vi "PS Control.vi"() -> ()   [LabVIEW 2025]
panel:
  in  "Stop":bool
  out "Tppms":dbl=378.0
  in  "set T":dbl=10.0
  in  "rate T":dbl=5.0 min=0.01 max=20.0
  in  "Setpoint [T]":dbl
  in  "Slew Rate [T/min]":dbl=0.3
  in  "T control":bool=TRUE
  in  "H control":bool=TRUE
  out "Field [T]":dbl=3.0
  out "helium level":bool
  out "LHe level":dbl=81.5
  out "error out":errorcluster
  out "Chamber\nStatus":i32(ring)=1 items=["ChamberUnknown"=0, "PurgedAndSealed"=1, "VentedAndSealed"=2, "Sealed"=3, "Purging"=4, "Venting"=5, "PreHiVac"=6, "HighVac"=7, "PumpContinuous"=8, "VentContinuous"=9, "ChamberFailure"=15]
  in  "set chamber":T1(ring)
  in  "shutdown":bool
  out "Field\nStatus":i32(ring)=4 items=["MagnetUnknown"=0, "StablePersistent"=1, "WarmingSwitch"=2, "CoolingSwitch"=3, "StableDriven"=4, "Iterating"=5, "Charging"=6, "Discharging"=7, "CurrentError"=8, "MagnetFailure"=15]
  out "Temperature\nStatus":i32(ring)=1 items=["TemperatureUnknown"=0, "Stable"=1, "Tracking"=2, "Near"=5, "Chasing"=6, "Filling"=7, "Standby"=10, "Disabled"=13, "ImpedanceNotFunction"=14, "TempFailure"=15]
  in  "LHe limit":dbl=60.0
  in  "resend chamber command":bool
  in  "Force High Vacuum":bool
  in  "HiVac pressure limit":dbl=0.0001 format="%#_4e"
  out "Position":dbl
  in  "Use rototar":bool
  in  "New position":dbl
  in  "Speed":dbl=5.0
  out "Pressure (Torr)":dbl=-1.0 format="%#_6e"
  in  "Mode":i32(ring) items=["Persistent", "Driven"]
  in  "Host (PPMS) computer name (or IP address)":string="SCM7"
  in  "port number":u16=3363
  # "(K/min)"
  # "Scroll down for a brief instruction."
  # "Error 56 or 63: Network error\n Possible reasons other than the obvious reasons (no internet, wrong host name, ...)\n   If the server program (PS Control.vi) is running under the development environment -> Check VI server settings (TCP/IP, port number, machine access).\n   If the server program is running under the run-time engine (.exe program) --> Check port number in the LV PPMS.ini file.\n  Try a different but similar port number.  \n Firewall issue on the host computer (rare) -> contact the computer support group.\n\nError 1004: server program not found (problem is at the host computer)\n Server program (PS Control.vi) is not running on the PPMS computer.  --> Start the server program.\n If the server program does not start, try to start it under a different mode (administrator or non-admininstrator). The server program will not start  unless it starts with the same mode with the PPMS multivu program.\n\nHow to use. \n\nFor  NML Data Acqustion.vi. (1) select 'Field' to read the field value, (2) select 'VI server read' to read the temperature (VI name: PS Control.vi, Control name: Tppms)\nFor LowMaster.vi, use the VI server menu to change the temperature, field and the other settings of the PPMS.\nFor MonoVu, use the built-in menu to control the field/temperature and the VI server menu to change the other settings of the PPMS."
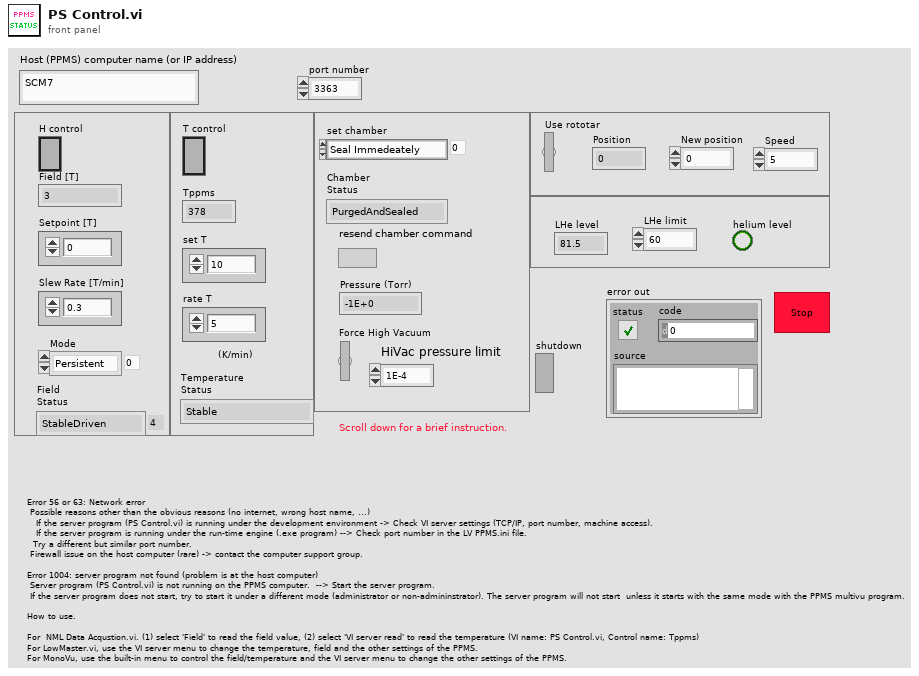
[diagram p1: front panel]
types:
  T1 = enum16{"Seal Immedeately", "Purge and Seal", "Vent and Seal", "Pump continuously", "Vent continuously", "HighVac"}
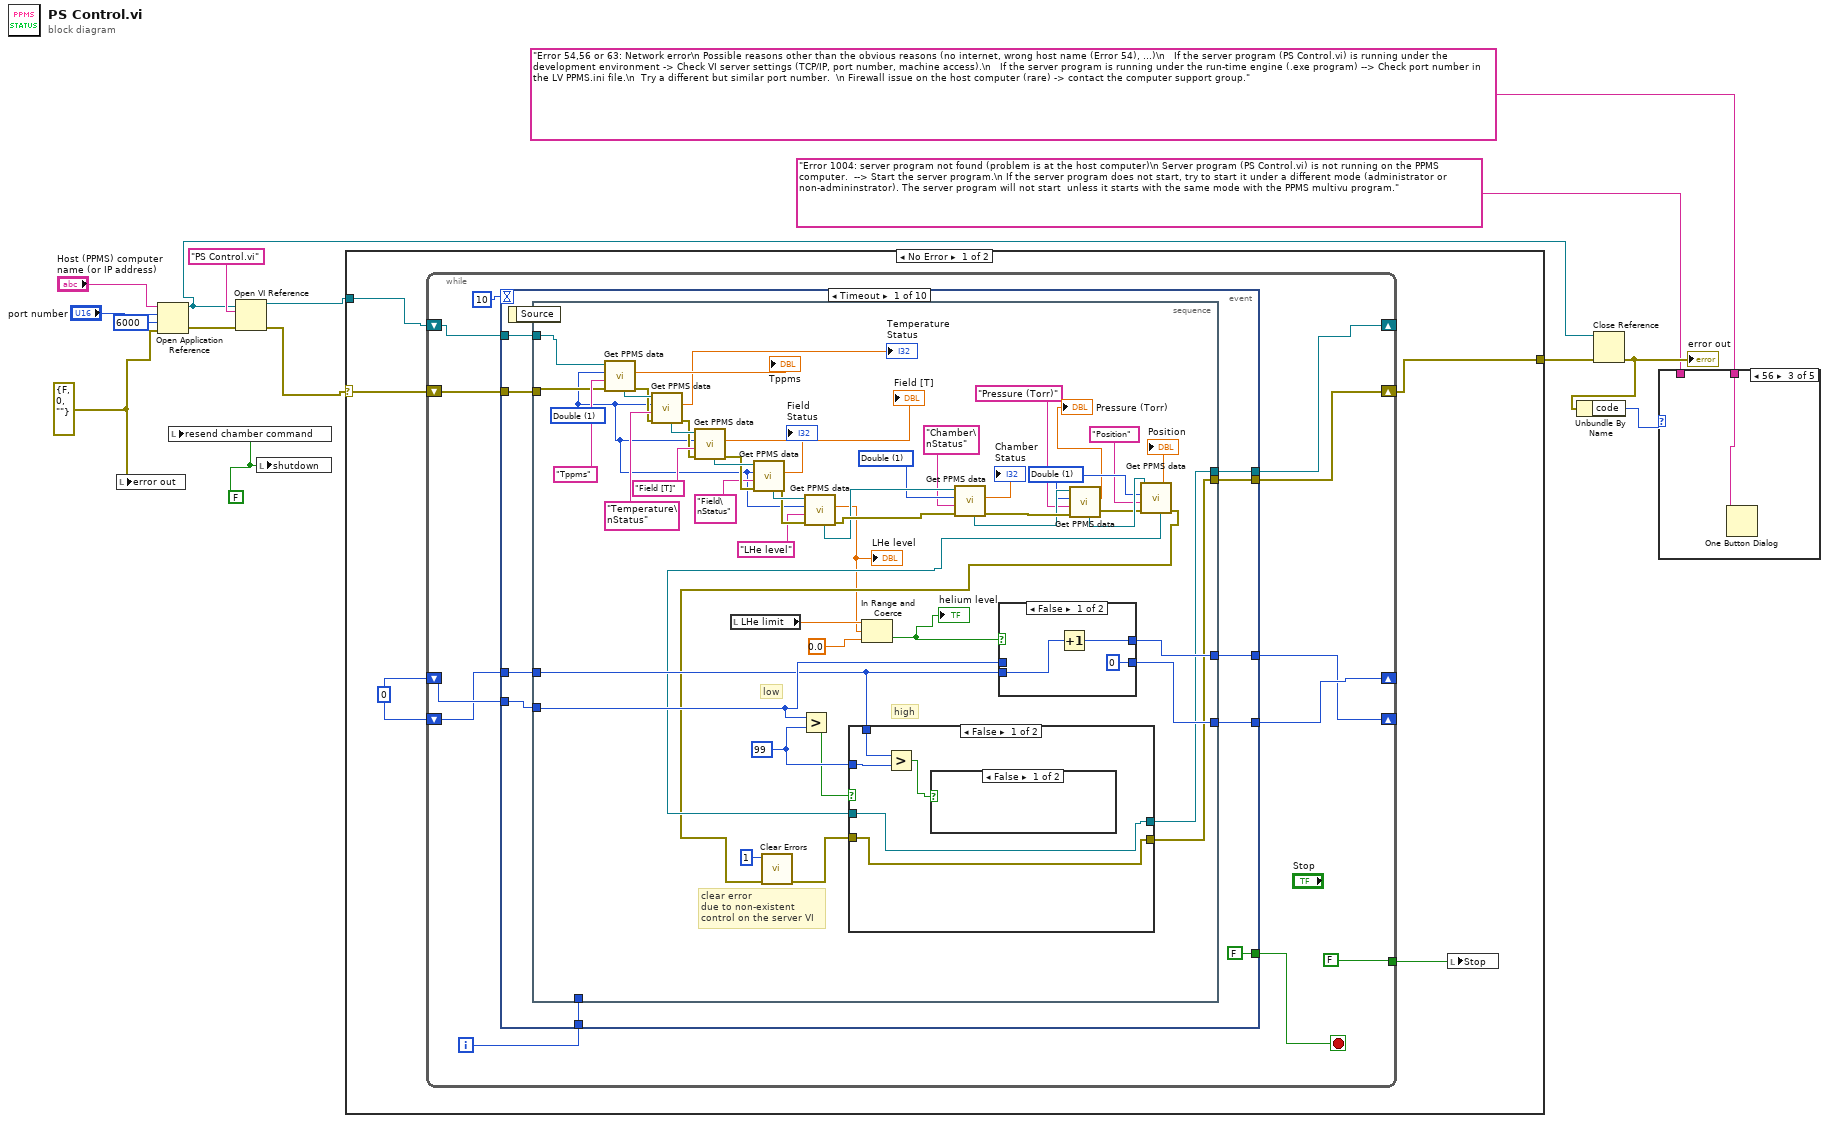
[diagram p0: block diagram]
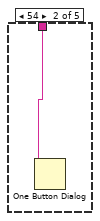
[diagram p3: hidden frame]
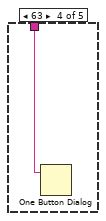
[diagram p4: hidden frame]
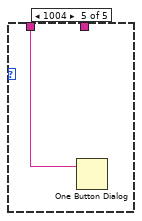
[diagram p5: hidden frame]
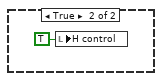
[diagram p6: hidden frame]
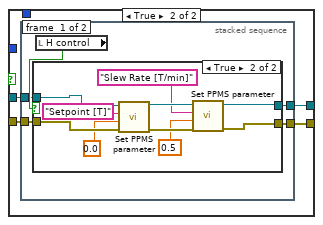
[diagram p7: hidden frame]
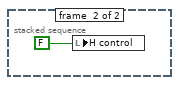
[diagram p9: hidden frame]
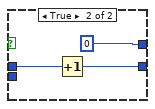
[diagram p10: hidden frame]
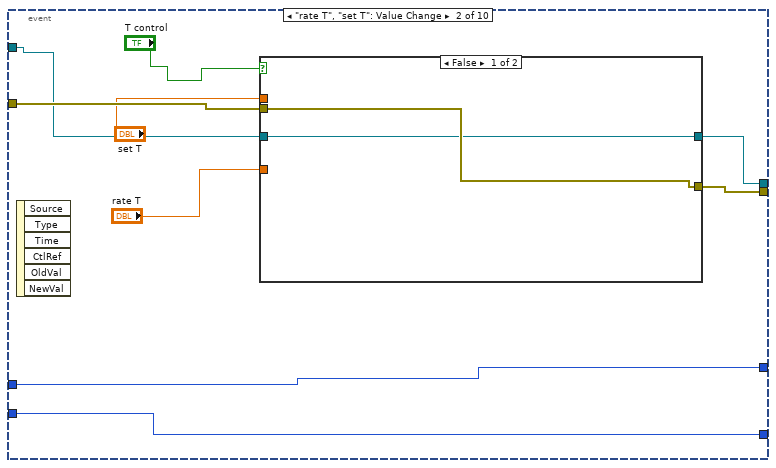
[diagram p11: hidden frame]
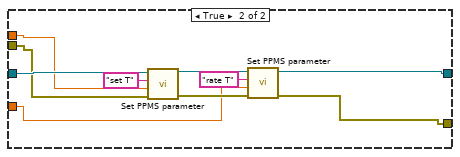
[diagram p12: hidden frame]
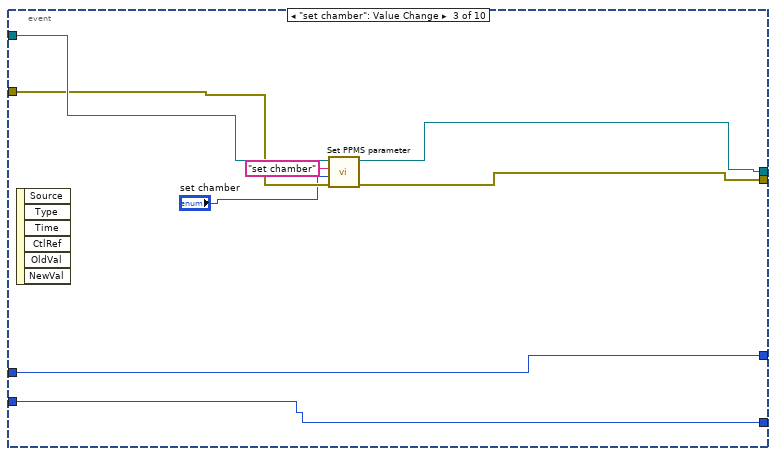
[diagram p13: hidden frame]
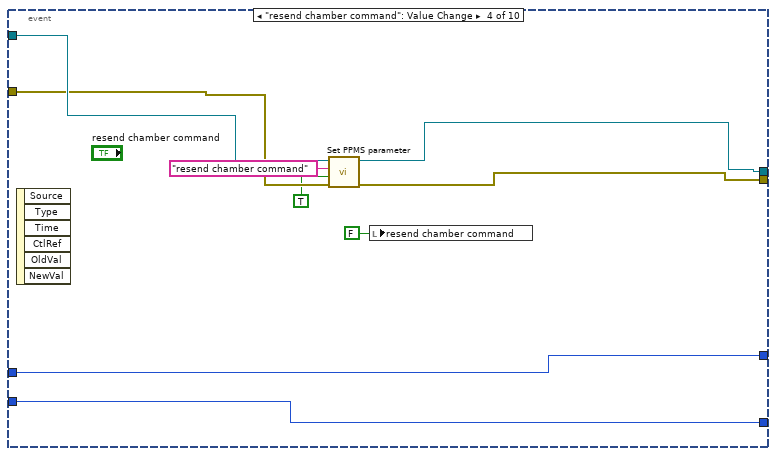
[diagram p14: hidden frame]
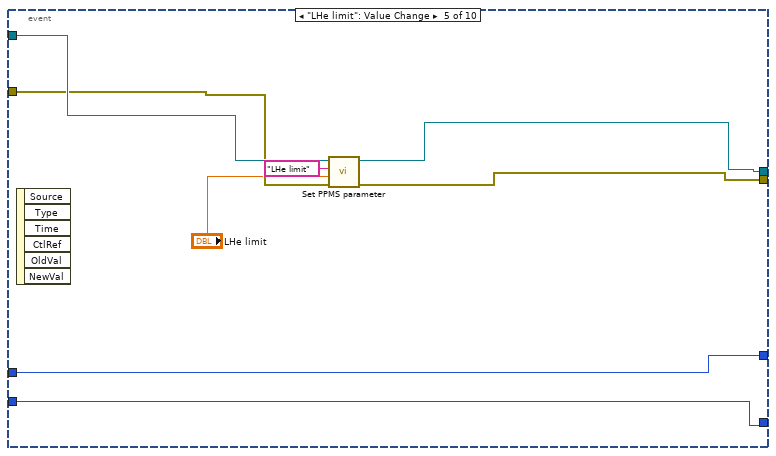
[diagram p15: hidden frame]
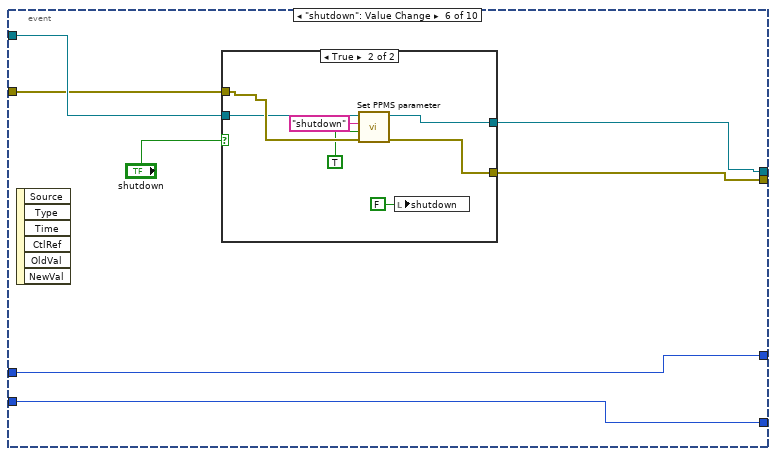
[diagram p16: hidden frame]
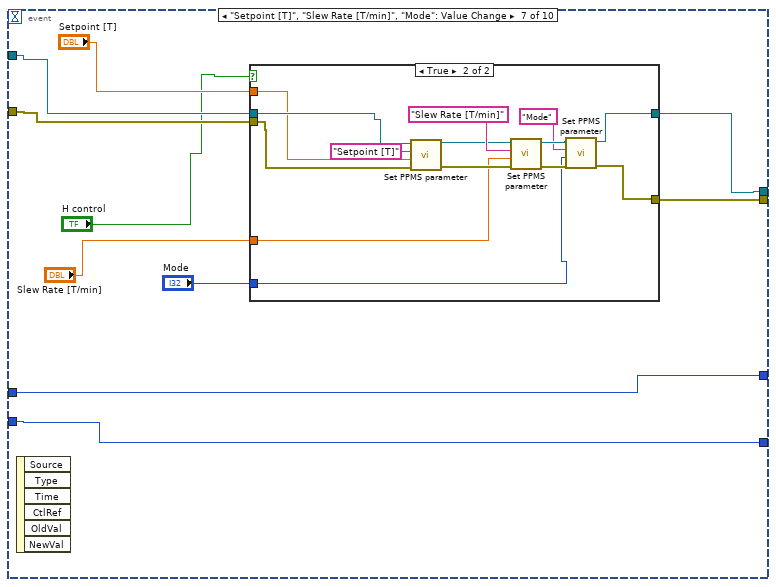
[diagram p18: hidden frame]
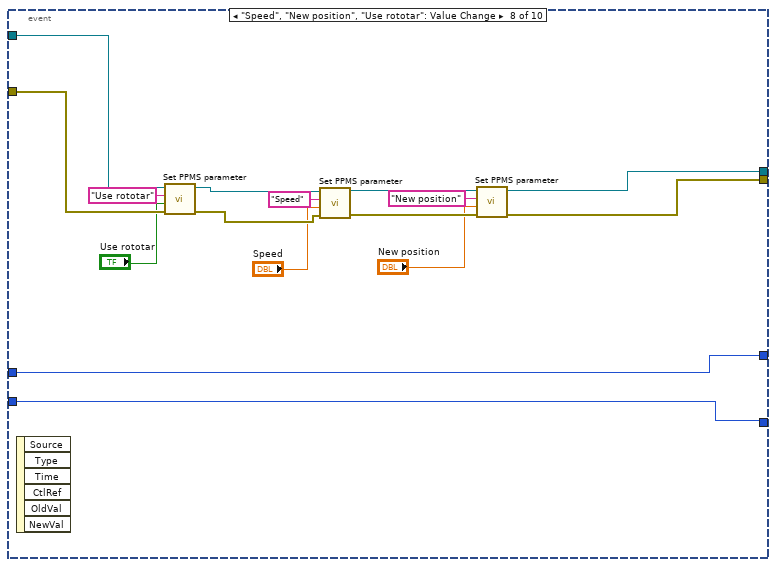
[diagram p20: hidden frame]
diagram:
  w5 = errorcluster {"status"=FALSE, "code"=0, "source"=""} ("error in (no error)")
  w8 = FALSE ("shutdown")
  n1 = local write "error out"(w5) -> ()
  n2 = Open Application Reference(8:w5, 9:6000 ("timeout ms (60000)"), 10:"port number", 11:"Host (PPMS) computer name (or IP address)") -> (0:w15:errorcluster, 3:w9:refnum<vi>)
  n3 = local write "resend chamber command"(w8) -> ()
  n4 = Open VI Reference(application reference (local)=w9, vi path="PS Control.vi" ("Machine Name 2"), error in (no error)=w15) -> (vi reference=w12:refnum<vi>, error out=w11:errorcluster)  [unwired: 3 in]
  n5 = local write "shutdown"(w8) -> ()
  n6 = case shown="No Error" w11 {
    selector: w11 -> [w20 w248]
    tunnel: w12 -> [w17 _]
    tunnel: [w16 w248] -> w7
    frame No Error {
      w18 = 0
      n7 = while {
        tunnel: [FALSE] -> w19
        shift-right: [w26] -> _
        shift-left: w18 -> [w27]
        shift-right: [w24] -> _
        shift-left: w18 -> [w25]
        shift-right: [w22] -> _
        shift-left: w17 -> [w23]
        shift-right: [w21] -> w16
        shift-left: w20 -> [w32]
        i -> [w28]
        stop <- w29 stop-if-true
        n8 = event shown="[0] Timeout" {
          selector: _ -> [_ _ _ _ _ _ _ _ _ _]
          dyn-events: _ -> [_ _ _ _ _ _ _ _ _ _]
          timeout: 10 -> [_ _ _ _ _ _ _ _ _ _]
          tunnel: w32 -> [w42 w134 w153 w162 w170 w178 w196 w222 w238 w246]
          tunnel: [FALSE ("NewVal") _ _ _ _ _ _ _ _ w247] -> w29
          tunnel: w28 -> [w40 _ _ _ _ _ _ _ _ _]
          tunnel: w27 -> [w39 w127 w148 w156 w165 w173 w189 w215 w231 w243]
          tunnel: [w38 w127 w148 w156 w165 w173 w189 w215 w231 w243] -> w26
          tunnel: w25 -> [w37 w128 w149 w157 w166 w174 w190 w216 w232 w244]
          tunnel: [w36 w128 w149 w157 w166 w174 w190 w216 w232 w244] -> w24
          tunnel: w23 -> [w35 w129 w155 w164 w172 w179 w198 w223 w237 w245]
          tunnel: [w34 w133 w154 w163 w171 w177 w197 w230 w233 w245] -> w22
          tunnel: [w33 w132 w152 w161 w169 w176 w195 w229 w234 w246] -> w21
          event Timeout {
            n9 = event-data() -> ()  [unwired: 1 in, 1 out]
            n10 = stacked-sequence {
              tunnel: w42 -> [w82]
              tunnel: w40 -> [_]
              tunnel: w39 -> [w91]
              tunnel: [w92] -> w38
              tunnel: w37 -> [w89]
              tunnel: [w90] -> w36
              tunnel: w35 -> [w85]
              tunnel: [w87] -> w34
              tunnel: [w86] -> w33
              frame #0 {
                w52 = u16 1 items=["String", "Double", "Boolean", "Variant"] ("Data Type")
                w63 = u16 1 items=["String", "Double", "Boolean", "Variant"] ("Data Type")
                w66 = u16 1 items=["String", "Double", "Boolean", "Variant"] ("Data Type")
                w88 = 99 ("y")
                # "clear error\ndue to non-existent\ncontrol on the server VI"
                # "high"
                # "low"
                n11 = call "Get PPMS data.vi"("error IO"=w82, "control"="Tppms", "Data Type"=w66, "vi reference"=w85) -> ("error out"=w74:errorcluster, "Data (Double)"=→"Tppms":dbl, "vi reference out"=w81:refnum<vi>)  [unwired: 2 in, 3 out]
                n12 = call "Get PPMS data.vi"("error IO"=w74, "control"="Temperature\nStatus", "Data Type"=w66, "vi reference"=w81) -> ("error out"=w73:errorcluster, "Data (Double)"=→"Temperature\nStatus":dbl, "vi reference out"=w78:refnum<vi>)  [unwired: 2 in, 3 out]
                n13 = call "Get PPMS data.vi"("error IO"=w73, "control"="Field [T]", "Data Type"=w66, "vi reference"=w78) -> ("error out"=w72:errorcluster, "Data (Double)"=→"Field [T]":dbl, "vi reference out"=w75:refnum<vi>)  [unwired: 2 in, 3 out]
                n14 = local read "LHe limit"() -> (w57:dbl)
                n15 = call "Get PPMS data.vi"("error IO"=w72, "control"="Field\nStatus", "Data Type"=w66, "vi reference"=w75) -> ("error out"=w68:errorcluster, "Data (Double)"=→"Field\nStatus":dbl, "vi reference out"=w69:refnum<vi>)  [unwired: 2 in, 3 out]
                n16 = Greater?(x=w91, y=w88) -> (0:w58:bool)
                n17 = call "Get PPMS data.vi"("error IO"=w68, "control"="LHe level", "Data Type"=w66, "vi reference"=w69) -> ("error out"=w65:errorcluster, "Data (Double)"=w43:dbl, "vi reference out"=w64:refnum<vi>)  [unwired: 2 in, 3 out]
                "LHe level" <- w43
                n18 = In Range and Coerce(upper limit=w57, x=w43, lower limit=0.0) -> (In Range?=w59:bool)  [unwired: 1 out]
                "helium level" <- w59
                n19 = call "Get PPMS data.vi"("error IO"=w65, "control"="Chamber\nStatus", "Data Type"=w63, "vi reference"=w64) -> ("error out"=w55:errorcluster, "Data (Double)"=→"Chamber\nStatus":dbl, "vi reference out"=w54:refnum<vi>)  [unwired: 2 in, 3 out]
                n20 = case shown="False" w59 {
                  tunnel: [0 w126] -> w92
                  tunnel: w91 -> [_ w125]
                  tunnel: w89 -> [w122 _]
                  tunnel: [w121 0 ("x+1")] -> w90
                  frame False {
                    n21 = Increment(x=w122) -> (x+1=w121:i32)
                  }
                  frame True {
                    n22 = Increment(x=w125) -> (x+1=w126:i32)
                  }
                }
                n23 = call "Get PPMS data.vi"("error IO"=w55, "control"="Pressure (Torr)", "Data Type"=w52, "vi reference"=w54) -> ("error out"=w47:errorcluster, "Data (Double)"=→"Pressure (Torr)":dbl, "vi reference out"=w53:refnum<vi>)  [unwired: 2 in, 3 out]
                n24 = call "Get PPMS data.vi"("error IO"=w47, "control"="Position", "Data Type"=w52, "vi reference"=w53) -> ("error out"=w46:errorcluster, "Data (Double)"=→"Position":dbl, "vi reference out"=w56:refnum<vi>)  [unwired: 2 in, 3 out]
                n25 = call <vilib>:"Clear Errors.vi"("error in (no error)"=w46, "specific error code to clear (0: all)"=1) -> ("error out"=w45:errorcluster)  [unwired: 4 in, 1 out]
                n26 = case shown="False" w58 {
                  tunnel: [w93 w102] -> w86
                  tunnel: w89 -> [w97 _]
                  tunnel: w88 -> [w96 _]
                  tunnel: w56 -> [w94 w101]
                  tunnel: [w94 w100] -> w87
                  tunnel: w45 -> [w93 w99]
                  frame False {
                    n27 = Greater?(x=w97, y=w96) -> (0:w95:bool)
                    n28 = case shown="False" w95 {
                      frame False {
                      }
                      frame True {
                        n29 = local write "H control"(TRUE ("H control")) -> ()
                      }
                    }
                  }
                  frame True {
                    n30 = stacked-sequence {
                      tunnel: [w107 _] -> w102
                      tunnel: w101 -> [w105 _]
                      tunnel: [w104 _] -> w100
                      tunnel: w99 -> [w103 _]
                      frame #0 {
                        n31 = local read "H control"() -> (w106:bool)
                        n32 = case shown="True" w106 {
                          tunnel: [w109 w115] -> w107
                          tunnel: w105 -> [w108 w119]
                          tunnel: [w108 w114] -> w104
                          tunnel: w103 -> [w109 w117]
                          frame False {
                          }
                          frame True {
                            n33 = call "Set PPMS parameter.vi"("error in (no error)"=w117, "Input Value"=0.0 ("Tppms"), "Control Name"="Setpoint [T]", "VI reference in"=w119) -> ("error out"=w116:errorcluster, "VI reference out"=w118:refnum<vi>)  [unwired: 6 in]
                            n34 = call "Set PPMS parameter.vi"("error in (no error)"=w116, "Input Value"=0.5 ("Tppms"), "Control Name"="Slew Rate [T/min]", "VI reference in"=w118) -> ("error out"=w115:errorcluster, "VI reference out"=w114:refnum<vi>)  [unwired: 6 in]
                          }
                        }
                      }
                      frame #1 {
                        n35 = local write "H control"(FALSE ("H control")) -> ()
                      }
                    }
                  }
                }
              }
            }
          }
          event "rate T", "set T": Value Change {
            n36 = event-data() -> ()  [unwired: 1 in, 6 out]
            n37 = case shown="False" "T control" {
              tunnel: "set T" -> [_ w144]
              tunnel: "rate T" -> [_ w141]
              tunnel: w134 -> [w137 w143]
              tunnel: [w136 w140] -> w133
              tunnel: [w137 w138] -> w132
              tunnel: w129 -> [w136 w147]
              frame False {
              }
              frame True {
                n38 = call "Set PPMS parameter.vi"("error in (no error)"=w143, "Input Value"=w144, "Control Name"="set T", "VI reference in"=w147) -> ("error out"=w142:errorcluster, "VI reference out"=w139:refnum<vi>)  [unwired: 6 in]
                n39 = call "Set PPMS parameter.vi"("error in (no error)"=w142, "Input Value"=w141, "Control Name"="rate T", "VI reference in"=w139) -> ("error out"=w138:errorcluster, "VI reference out"=w140:refnum<vi>)  [unwired: 6 in]
              }
            }
          }
          event "set chamber": Value Change {
            n40 = event-data() -> ()  [unwired: 1 in, 6 out]
            n41 = call "Set PPMS parameter.vi"("error in (no error)"=w153, "Input Value"="set chamber", "Control Name"="set chamber", "VI reference in"=w155) -> ("error out"=w152:errorcluster, "VI reference out"=w154:refnum<vi>)  [unwired: 6 in]
          }
          event "resend chamber command": Value Change {
            n42 = event-data() -> ()  [unwired: 1 in, 6 out]
            n43 = call "Set PPMS parameter.vi"("error in (no error)"=w162, "Input Value"=TRUE ("resend chamber command"), "Control Name"="resend chamber command", "VI reference in"=w164) -> ("error out"=w161:errorcluster, "VI reference out"=w163:refnum<vi>)  [unwired: 6 in]
            n44 = local write "resend chamber command"(FALSE ("resend chamber command")) -> ()
          }
          event "LHe limit": Value Change {
            n45 = event-data() -> ()  [unwired: 1 in, 6 out]
            n46 = call "Set PPMS parameter.vi"("error in (no error)"=w170, "Input Value"="LHe limit", "Control Name"="LHe limit", "VI reference in"=w172) -> ("error out"=w169:errorcluster, "VI reference out"=w171:refnum<vi>)  [unwired: 6 in]
          }
          event "shutdown": Value Change {
            n47 = event-data() -> ()  [unwired: 1 in, 6 out]
            n48 = case shown="True" "shutdown" {
              tunnel: w179 -> [w180 w185]
              tunnel: w178 -> [w181 w186]
              tunnel: [w180 w184] -> w177
              tunnel: [w181 w183] -> w176
              frame False {
              }
              frame True {
                n49 = call "Set PPMS parameter.vi"("error in (no error)"=w186, "Input Value"=TRUE ("shutdown"), "Control Name"="shutdown", "VI reference in"=w185) -> ("error out"=w183:errorcluster, "VI reference out"=w184:refnum<vi>)  [unwired: 6 in]
                n50 = local write "shutdown"(FALSE ("shutdown")) -> ()
              }
            }
          }
          event "Setpoint [T]", "Slew Rate [T/min]", "Mode": Value Change {
            n51 = event-data() -> ()  [unwired: 1 in, 6 out]
            n52 = case shown="True" "H control" {
              tunnel: w198 -> [w200 w209]
              tunnel: [w200 w205] -> w197
              tunnel: w196 -> [w199 w210]
              tunnel: [w199 w203] -> w195
              tunnel: "Setpoint [T]" -> [_ w208]
              tunnel: "Slew Rate [T/min]" -> [_ w207]
              tunnel: "Mode" -> [_ w201]
              frame False {
              }
              frame True {
                n53 = call "Set PPMS parameter.vi"("error in (no error)"=w210, "Input Value"=w208, "Control Name"="Setpoint [T]", "VI reference in"=w209) -> ("error out"=w212:errorcluster, "VI reference out"=w211:refnum<vi>)  [unwired: 6 in]
                n54 = call "Set PPMS parameter.vi"("error in (no error)"=w212, "Input Value"=w207, "Control Name"="Slew Rate [T/min]", "VI reference in"=w211) -> ("error out"=w204:errorcluster, "VI reference out"=w206:refnum<vi>)  [unwired: 6 in]
                n55 = call "Set PPMS parameter.vi"("error in (no error)"=w204, "Input Value"=w201, "Control Name"="Mode", "VI reference in"=w206) -> ("error out"=w203:errorcluster, "VI reference out"=w205:refnum<vi>)  [unwired: 6 in]
              }
            }
          }
          event "Speed", "New position", "Use rototar": Value Change {
            n56 = event-data() -> ()  [unwired: 1 in, 6 out]
            n57 = call "Set PPMS parameter.vi"("error in (no error)"=w222, "Input Value"="Use rototar", "Control Name"="Use rototar", "VI reference in"=w223) -> ("error out"=w219:errorcluster, "VI reference out"=w224:refnum<vi>)  [unwired: 6 in]
            n58 = call "Set PPMS parameter.vi"("error in (no error)"=w219, "Input Value"="Speed", "Control Name"="Speed", "VI reference in"=w224) -> ("error out"=w226:errorcluster, "VI reference out"=w225:refnum<vi>)  [unwired: 6 in]
            n59 = call "Set PPMS parameter.vi"("error in (no error)"=w226, "Input Value"="New position", "Control Name"="New position", "VI reference in"=w225) -> ("error out"=w229:errorcluster, "VI reference out"=w230:refnum<vi>)  [unwired: 6 in]
          }
          event "HiVac pressure limit", "Force High Vacuum": Value Change {
            n60 = event-data() -> ()  [unwired: 1 in, 6 out]
            n61 = call "Set PPMS parameter.vi"("error in (no error)"=w238, "Input Value"="Force High Vacuum", "Control Name"="Force High Vacuum", "VI reference in"=w237) -> ("error out"=w239:errorcluster, "VI reference out"=w241:refnum<vi>)  [unwired: 6 in]
            n62 = call "Set PPMS parameter.vi"("error in (no error)"=w239, "Input Value"="HiVac pressure limit", "Control Name"="HiVac pressure limit", "VI reference in"=w241) -> ("error out"=w234:errorcluster, "VI reference out"=w233:refnum<vi>)  [unwired: 6 in]
          }
          event "Stop": Value Change {
            n63 = event-data() -> ("NewVal"=w247:bool)  [unwired: 1 in]
          }
        }
      }
      n64 = local write "Stop"(w19) -> ()
    }
    frame Error {
    }
  }
  n65 = Close Reference(reference=w9, error in (no error)=w7) -> (error out=w4:errorcluster)
  "error out" <- w4
  n66 = Unbundle By Name(w4) -> ("code"=w3:i32)
  n67 = case shown="56" w3 {
    tunnel: "Error 1004: server program not found (problem is at the host computer)\n Server program (PS Control.vi) is not running on the PPMS computer.  --> Start the server program.\n If the server program does not start, try to start it under a different mode (administrator or non-admininstrator). The server program will not start  unless it starts with the same mode with the PPMS multivu program." ("message") -> [_ _ _ _ w252]
    tunnel: "Error 54,56 or 63: Network error\n Possible reasons other than the obvious reasons (no internet, wrong host name (Error 54), ...)\n   If the server program (PS Control.vi) is running under the development environment -> Check VI server settings (TCP/IP, port number, machine access).\n   If the server program is running under the run-time engine (.exe program) --> Check port number in the LV PPMS.ini file.\n  Try a different but similar port number.  \n Firewall issue on the host computer (rare) -> contact the computer support group." ("message") -> [_ w249 w250 w251 _]
    frame 0, Default {
    }
    frame 54 {
      n68 = One Button Dialog(message=w249) -> ()  [unwired: 1 in, 1 out]
    }
    frame 56 {
      n69 = One Button Dialog(message=w250) -> ()  [unwired: 1 in, 1 out]
    }
    frame 63 {
      n70 = One Button Dialog(message=w251) -> ()  [unwired: 1 in, 1 out]
    }
    frame 1004 {
      n71 = One Button Dialog(message=w252) -> ()  [unwired: 1 in, 1 out]
    }
  }
